vi "CLD 8 CSV file commands utility Exercise.vi"(8 "Error In":errorcluster) -> (0 "Error Out":errorcluster, 3 "Commands Out Array":T1[](array[typedef]))   [LabVIEW 2009]
doc: "CLD 8 exercise"
uses:
  CLD 8 Data Cluster.ctl
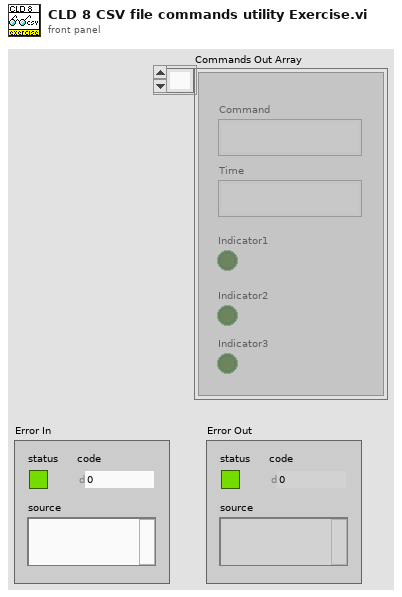
[diagram p1: front panel]
types:
  T1 = typedef "CLD 8 Data Cluster.ctl" = cluster{"Command":string, "Time":string, "Indicator1":bool, "Indicator2":bool, "Indicator3":bool}
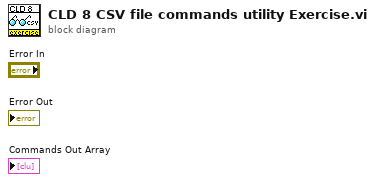
[diagram p0: block diagram]
diagram:
